vi "Configure_Voltage_Level.vi"(8 "error in (no error)":errorcluster, 10 "Level":dbl=1.2, 11 "NI-DCPower in":refnum<class "niDCPower.lvclass">) -> (0 "error out":errorcluster, 3 "NI-DCPower out":refnum<class "niDCPower.lvclass">)   [LabVIEW 2021, in "niDCPower.lvclass"]
uses:
  niDCPower.lvclass
  niDCPower.lvclass/niDCPower.ctl
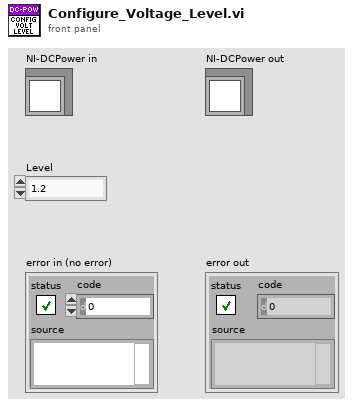
[diagram p1: front panel]
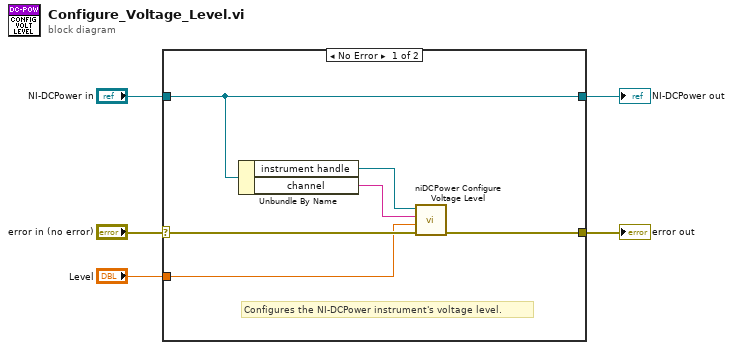
[diagram p0: block diagram]
diagram:
  n1 = case shown="No Error" "error in (no error)" {
    selector: "error in (no error)" -> [w11 w13]
    tunnel: [w10 w13] -> w4
    tunnel: [w9 w12] -> w2
    tunnel: "NI-DCPower in" -> [w9 w12]
    tunnel: "Level" -> [w6 _]
    frame No Error {
      # "Configures the NI-DCPower instrument's voltage level."
      n2 = Unbundle By Name(w9) -> ("instrument handle"=w8:refnum<k15>, "channel"=w7:string)
      n3 = call <instrlib>:"niDCPower Configure Voltage Level.vi"("error in (no error)"=w11, "voltage level"=w6, "channel name"=w7, "instrument handle"=w8) -> ("error out"=w10:errorcluster)  [unwired: 6 in, 1 out]
    }
    frame Error {
    }
  }
  "error out" <- w4
  "NI-DCPower out" <- w2
